vi "INI_34465A.vi"(5 "MCListbox Ref":refnum<vi>, 9 "MListBox Row":u16=2 max=8, 11 "Device INI Config File Path":path=path "D:/LABVIEW/Examples/INI Devices/DeviceConfig.ini") -> (0 "error out":errorcluster, 3 "Serial_VISA":T1)   [LabVIEW 2018]
uses:
  Examples - 32bit/SEQUENCER/SEQUENSER v10/Sequencer v10/Ctl/Serial_VISA.ctl
  <vilib>/Utility/miscctls.llb/LVRowAndColumnTypeDef.ctl
  <vilib>/Utility/config.llb/Read Key (String).vi
  <vilib>/Utility/config.llb/NI_LVConfig.lvlib
  <instrlib>/Agilent 3446X Series/Agilent 3446X Series.lvlib
panel:
  out "Array DMM":string[](array[string])
  out "DMM Read Buffer":string
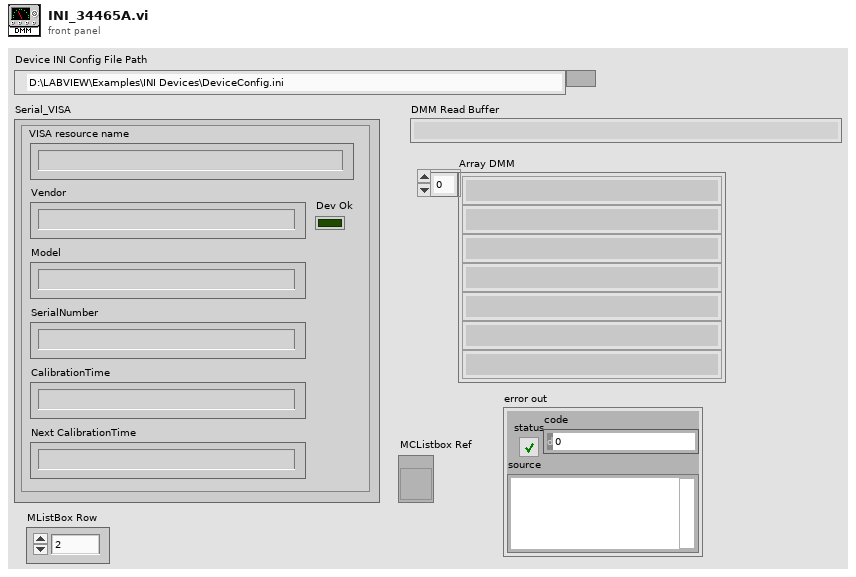
[diagram p1: front panel]
types:
  T1 = typedef "Serial_VISA.ctl" = cluster{"VISA resource name":string, "Vendor":string, "SerialNumber":string, "CalibrationTime":string, "Dev Ok":bool, "Model":string, "Next CalibrationTime":string}
  T2 = typedef "LVRowAndColumnTypeDef.ctl" = cluster{"Row":i32, "Column":i32}
  T3 = typedef "NI_LVConfig.lvlib/Config Data RefNum.ctl" = refnum<k1>
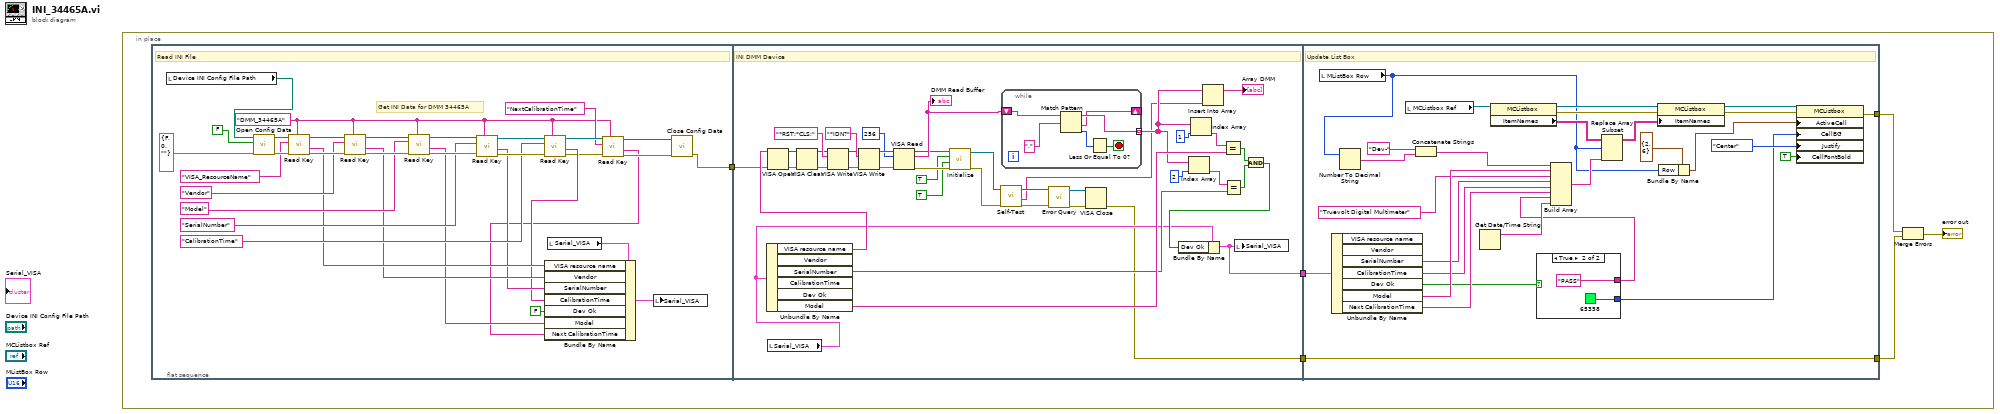
[diagram p0: block diagram]
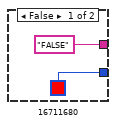
[diagram p2: hidden frame]
diagram:
  n1 = in-place {
    n2 = flat-sequence {
      tunnel: [w8] -> w6
      tunnel: w6 -> [w43]
      tunnel: [w42] -> w4
      tunnel: [w41] -> w1
      tunnel: [w93] -> w5
      tunnel: [w92] -> w3
      tunnel: w4 -> [w92]
      tunnel: w1 -> [w90]
      frame #0 {
        w13 = "DMM_34465A" ("section")
        # "Get INI Data for DMM 34465A"
        # "Read INI File"
        n3 = local read "Device INI Config File Path"() -> (w7:path)
        n4 = call <vilib>:"Open Config Data.vi"("error in (no error)"=errorcluster {"status"=FALSE, "code"=0, "source"=""} ("error constant"), "create file if necessary (T)"=FALSE, "configuration file path"=w7) -> ("error out"=w38:errorcluster, "refnum"=w39:T3)  [unwired: 6 in, 1 out]
        n5 = call-poly <vilib>:"Read Key.vi"("section"=w13, "error in (no error)"=w38, "key"="VISA_ResourceName", "refnum"=w39) -> ("error out"=w35:errorcluster, "value"=w24:string, "refnum out"=w37:T3)  [unwired: 4 in, 1 out]
        n6 = call-poly <vilib>:"Read Key.vi"("section"=w13, "error in (no error)"=w35, "key"="Vendor", "refnum"=w37) -> ("error out"=w34:errorcluster, "value"=w23:string, "refnum out"=w36:T3)  [unwired: 4 in, 1 out]
        n7 = call-poly <vilib>:"Read Key.vi"("section"=w13, "error in (no error)"=w34, "key"="Model", "refnum"=w36) -> ("error out"=w29:errorcluster, "value"=w22:string, "refnum out"=w30:T3)  [unwired: 4 in, 1 out]
        n8 = call-poly <vilib>:"Read Key.vi"("section"=w13, "error in (no error)"=w29, "key"="SerialNumber", "refnum"=w30) -> ("error out"=w26:errorcluster, "value"=w21:string, "refnum out"=w27:T3)  [unwired: 4 in, 1 out]
        n9 = call-poly <vilib>:"Read Key.vi"("section"=w13, "error in (no error)"=w26, "key"="CalibrationTime", "refnum"=w27) -> ("error out"=w17:errorcluster, "value"=w20:string, "refnum out"=w18:T3)  [unwired: 4 in, 1 out]
        n10 = local read "Serial_VISA"() -> (w10:T1)
        n11 = call-poly <vilib>:"Read Key.vi"("section"=w13, "error in (no error)"=w17, "key"="NextCalibrationTime", "refnum"=w18) -> ("error out"=w15:errorcluster, "value"=w12:string, "refnum out"=w16:T3)  [unwired: 4 in, 1 out]
        n12 = Bundle By Name(cluster=w10, "VISA resource name"=w24, "Vendor"=w23, "SerialNumber"=w21, "CalibrationTime"=w20, "Dev Ok"=FALSE, "Model"=w22, "Next CalibrationTime"=w12) -> (w9:T1)
        n13 = local write "Serial_VISA"(w9) -> ()
        n14 = call <vilib>:"Close Config Data.vi"("error in (no error)"=w15, "refnum"=w16) -> ("error out"=w8:errorcluster)  [unwired: 8 in, 1 out]
      }
      frame #1 {
        # "INI DMM Device"
        n15 = local read "Serial_VISA"() -> (w44:T1)
        n16 = Unbundle By Name(w44) -> ("VISA resource name"=w68:string, "SerialNumber"=w61:string, "Model"=w64:string)  [unwired: 3 out]
        n17 = VISA Open(error in (no error)=w43, VISA resource name=w68) -> (VISA resource name=w71:refnum<visa-resource-name>, error out=w70:errorcluster)  [unwired: 3 in]
        n18 = VISA Clear(VISA resource name=w71, error in (no error)=w70) -> (VISA resource name out=w72:refnum<visa-resource-name>, error out=w69:errorcluster)
        n19 = VISA Write(VISA resource name=w72, write buffer="*RST;*CLS;", error in (no error)=w69) -> (VISA resource name out=w74:refnum<visa-resource-name>, error out=w73:errorcluster)  [unwired: 1 out]
        n20 = VISA Write(VISA resource name=w74, write buffer="*IDN?", error in (no error)=w73) -> (VISA resource name out=w78:refnum<visa-resource-name>, error out=w77:errorcluster)  [unwired: 1 out]
        n21 = VISA Read(VISA resource name=w78, byte count=u32 256, error in (no error)=w77) -> (VISA resource name out=w57:refnum<visa-resource-name>, read buffer=w67:string, error out=w56:errorcluster)  [unwired: 1 out]
        "DMM Read Buffer" <- w67
        n22 = call <instrlib>:"Initialize.vi"("error in (no error)"=w56, "Reset (True)"=TRUE, "ID Query (True)"=TRUE, "VISA resource name"=w57) -> ("error out"=w48:errorcluster, "VISA resource name out"=w49:refnum<visa-resource-name>)  [unwired: 6 in]
        n23 = call <instrlib>:"Self-Test.vi"("error in (no error)"=w48, "VISA resource name"=w49) -> ("error out"=w50:errorcluster, "Self-Test Result Message"=w45:string, "VISA resource name out"=w52:refnum<visa-resource-name>)  [unwired: 6 in, 1 out]
        n24 = while {
          shift-right: [w82] -> _
          shift-left: w67 -> [w85]
          tunnel: [w83] -> w47 mode=indexing
          stop <- w80 stop-if-true
          n25 = Match Pattern(string=w85, regular expression="," ("search string/char (-)")) -> (before substring=w83:string, after substring=w82:string, offset past match=w81:i32)  [unwired: 1 in, 1 out]
          n26 = Less Or Equal To 0?(x=w81) -> (x <= 0?=w80:bool)
        }
        n27 = call <instrlib>:"Error Query.vi"("error in (no error)"=w50, "VISA resource name"=w52) -> ("error out"=w51:errorcluster, "VISA resource name out"=w53:refnum<visa-resource-name>)  [unwired: 8 out]
        n28 = VISA Close(VISA resource name=w53, error in (no error)=w51) -> (error out=w42:errorcluster)
        n29 = Index Array(array=w47, index=2) -> (element=w63:string)
        n30 = Index Array(array=w47, index=1) -> (element=w65:string)
        n31 = Insert Into Array(array=w47, new element=w45) -> (→"Array DMM":string[])  [unwired: 1 in]
        n32 = Equal?(x=w65, y=w64) -> (x = y?=w60:bool)
        n33 = Equal?(x=w63, y=w61) -> (x = y?=w59:bool)
        n34 = And(x=w60, y=w59) -> (x .and. y?=w58:bool)
        n35 = Bundle By Name(cluster=w44, "Dev Ok"=w58) -> (w41:T1)
        n36 = local write "Serial_VISA"(w41) -> ()
      }
      frame #2 {
        # "Update List Box"
        n37 = local read "MListBox Row"() -> (w87:u16)
        n38 = Unbundle By Name(w90) -> ("SerialNumber"=w110:string, "CalibrationTime"=w111:string, "Dev Ok"=w96:bool, "Model"=w112:string, "Next CalibrationTime"=w113:string)  [unwired: 2 out]
        n39 = Number To Decimal String(number=w87) -> (decimal integer string=w89:string)  [unwired: 1 in]
        n40 = local read "MCListbox Ref"() -> (w100:refnum<vi>)
        n41 = Concatenate Strings("Dev-", w89) -> (w86:string)
        n42 = Get Date/Time String() -> (date string=w99:string)  [unwired: 3 in, 1 out]
        n43 = property class="MCListbox"(reference=w100) -> (reference out=w103:refnum<vi>, error out=w104:errorcluster, "ItemNames"=w105:string[][])  [unwired: 1 in]
        n44 = case shown="True" w96 {
          tunnel: [u32 16711680 u32 65358] -> w95
          tunnel: ["FALSE" ("element") "PASS" ("element")] -> w94
          frame False {
          }
          frame True {
          }
        }
        n45 = Build Array(w86, w112, "Truevolt Digital Multimeter", w110, w111, w113, w94, w99) -> (w107:string[])
        n46 = Replace Array Subset(array=w105, new element=w107, index (row)=w87) -> (w106:string[][])  [unwired: 1 in]
        n47 = property class="MCListbox"(reference=w103, error in=w104, "ItemNames"=w106) -> (reference out=w108:refnum<vi>, error out=w109:errorcluster)
        n48 = Bundle By Name(cluster=T2 {"Row"=2, "Column"=6} ("Active Cell:Active Cell"), "Row"=w87) -> (w97:T2)
        n49 = property class="MCListbox"(reference=w108, error in=w109, "ActiveCell"=w97, "CellBG"=w95, "Justify"=enum16{"Left", "Center", "Right"}."Center" ("Active Cell:Cell Justification"), "CellFontBold"=TRUE ("Active Cell:Cell Font:Bold")) -> (error out=w93:errorcluster)  [unwired: 1 out]
      }
    }
    n50 = Merge Errors(w5, w3) -> (→"error out":errorcluster)
  }
